vi "Seek.vi"(5 "Username":string, 6 "Password":string, 7 "Address":string, 8 "Error In":errorcluster) -> (0 "Error Out":errorcluster)   [LabVIEW 2018, in "Tests.lvlib" / "SFTP File.lvlib"]
uses:
  SFTP File.lvlib
  src/Toolkit/API/SFTP File/API/Typedefs/Flags.ctl
  <vilib>/addons/_JKI Toolkits/Caraya/classes/Test/Test.lvclass
  <vilib>/addons/_JKI Toolkits/Caraya/classes/Assert/Assert.lvclass
  src/Toolkit/API/SFTP File/SFTP File.lvclass
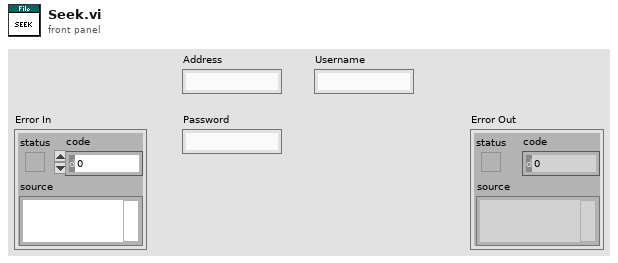
[diagram p1: front panel]
types:
  T1 = typedef "Toolkit.lvlib/SFTP File.lvclass/Flags.ctl" = cluster{"Read":bool, "Write":bool, "Append":bool, "Create":bool, "Truncate":bool, "Exclude":bool}
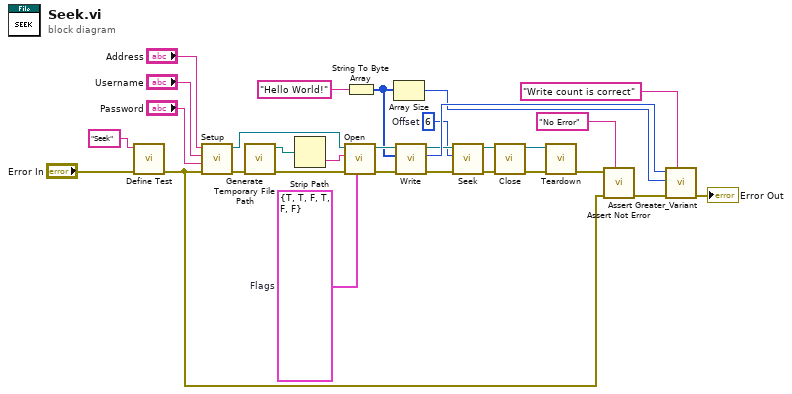
[diagram p0: block diagram]
diagram:
  w1 = u64 6  # Offset
  w6 = T1 {"Read"=TRUE, "Write"=TRUE, "Append"=FALSE, "Create"=TRUE, "Truncate"=FALSE, "Exclude"=FALSE}  # Flags
  n1 = call <vilib>:"Define Test.vi"("error in (no error)"="Error In", "Label (VI Title)"="Seek") -> ("error out"=w21:errorcluster)  [unwired: 9 in]
  n2 = call "Setup.vi"("Error In"=w21, "Password"="Password", "Username"="Username", "Address"="Address") -> ("Error Out"=w16:errorcluster, "SFTP"=w18:refnum<class "SFTP.lvclass">)  [unwired: 6 in]
  n3 = call <vilib>:"Generate Temporary File Path.vi"("error in (no error)"=w16) -> ("error out"=w15:errorcluster, "Unique Temporary File Path"=w14:path)  [unwired: 9 in]
  n4 = Strip Path(path=w14) -> (name=w13:string)  [unwired: 1 out]
  n5 = call "Open.vi"("Flags"=w6, "Error In"=w15, "Remote Path"=w13, "SFTP"=w18) -> ("Error Out"=w10:errorcluster, "SFTP File"=w12:refnum<class "SFTP File.lvclass">)  [unwired: 6 in]
  n6 = String To Byte Array(string="Hello World!") -> (unsigned byte array=w8:u8[])
  n7 = Array Size(array=w8) -> (size(s)=w7:i32)
  n8 = call "Write.vi"("Error In"=w10, "Data"=w8, "SFTP File In"=w12) -> ("Error Out"=w4:errorcluster, "Count"=w11:i64, "SFTP File Out"=w5:refnum<class "SFTP File.lvclass">)  [unwired: 6 in]
  n9 = call "Seek.vi"("Error In"=w4, "Offset"=w1, "SFTP File In"=w5) -> ("Error Out"=w3:errorcluster, "SFTP File Out"=w2:refnum<class "SFTP File.lvclass">)  [unwired: 7 in]
  n10 = call "Close.vi"("Error In"=w3, "SFTP File"=w2) -> ("Error Out"=w20:errorcluster, "SFTP"=w17:refnum<class "SFTP.lvclass">)  [unwired: 8 in]
  n11 = call "Teardown.vi"("Error In"=w20, "SFTP"=w17) -> ("Error Out"=w19:errorcluster)  [unwired: 9 in]
  n12 = call <vilib>:"Assert Not Error.vi"("Label"="No Error", "error in (no error)"=w21, "Not Error?"=w19) -> ("error out"=w27:errorcluster)  [unwired: 8 in]
  n13 = call <vilib>:"Assert Greater_Variant.vi"("Label"="Write count is correct", "error in (no error)"=w27, "Y"=w7, "X"=w11) -> ("error out"=→"Error Out":errorcluster)  [unwired: 7 in]
